vi "Execute.vi"(5 "Init user event out":refnum<user-event>, 7 "user event in":refnum<user-event>, 8 "Advanced Waveform In":refnum<class "Advanced Waveform.lvclass">, 9 "Generate From File in":refnum<class "Generate From File.lvclass">, 10 "Command Queue":refnum<queue>, 11 "error in (no error)":errorcluster) -> (0 "Advanced Waveform Out":refnum<class "Advanced Waveform.lvclass">, 1 "Generate From File Out":refnum<class "Generate From File.lvclass">, 2 "Stop":bool, 3 "error out":errorcluster)   [LabVIEW 2011, in "Generate From File.lvclass"]
uses:
  Generate From File.lvclass
  Advanced Waveform Class/Advanced Waveform.lvclass
  Message.lvclass
  Generate Class/Generate.lvclass
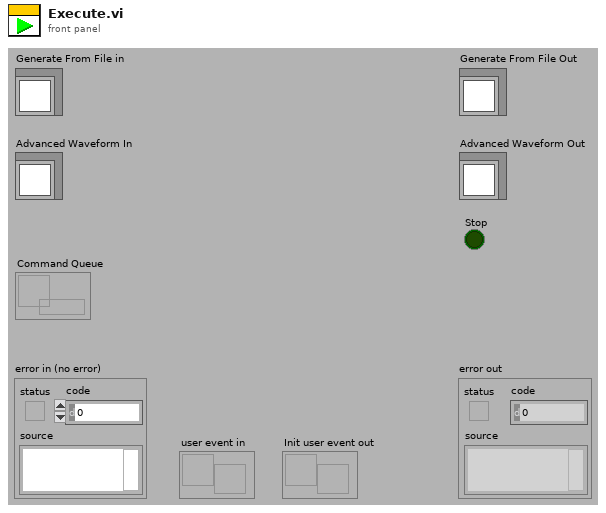
[diagram p1: front panel]
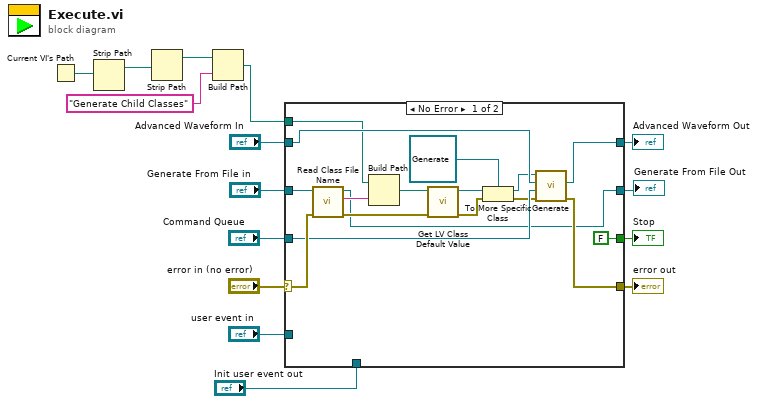
[diagram p0: block diagram]
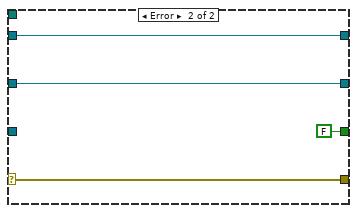
[diagram p2: hidden frame]
diagram:
  n1 = Current VI's Path() -> (path=w11:path)
  n2 = Strip Path(path=w11) -> (stripped path=w10:path)  [unwired: 1 out]
  n3 = Strip Path(path=w10) -> (stripped path=w9:path)  [unwired: 1 out]
  n4 = Build Path(base path=w9, name or relative path="Generate Child Classes") -> (appended path=w7:path)
  n5 = case shown="No Error" "error in (no error)" {
    selector: "error in (no error)" -> [w31 w35]
    tunnel: "Command Queue" -> [w26 _]
    tunnel: "Generate From File in" -> [w32 w33]
    tunnel: "Advanced Waveform In" -> [w28 w36]
    tunnel: w7 -> [w17 _]
    tunnel: [w27 w36] -> w6
    tunnel: [FALSE FALSE] -> w5
    tunnel: [w24 w35] -> w4
    tunnel: [w18 w33] -> w3
    tunnel: "user event in" -> [_ _]
    tunnel: "Init user event out" -> [_ _]
    frame No Error {
      n6 = call-dynamic "Read Class File Name.vi"("error in (no error)"=w31, "Generate From File in"=w32) -> ("error out"=w29:errorcluster, "Class File Name"=w30:string, "Generate From File out"=w18:refnum<class "Generate From File.lvclass">)  [unwired: 7 in]
      n7 = Build Path(base path=w17, name or relative path=w30) -> (appended path=w16:path)
      n8 = call <vilib>:"Get LV Class Default Value.vi"("error in (no error)"=w29, "class path"=w16) -> ("error out"=w22:errorcluster, "object"=w23:refnum<class>)  [unwired: 8 in]
      n9 = To More Specific Class(target class=refnum<class "Generate.lvclass"> refnum ("Generate.lvclass"), reference=w23, error in=w22) -> (specific class reference=w20:refnum<class "Generate.lvclass">, error out=w21:errorcluster)
      n10 = call-dynamic "Generate.vi"("error in (no error)"=w21, "Message Queue"=w26, "Advanced Waveform.lvclass In"=w28, "Generate in"=w20) -> ("error out"=w24:errorcluster, "Advanced Waveform.lvclass Out"=w27:refnum<class "Advanced Waveform.lvclass">)  [unwired: 4 in, 2 out]
    }
    frame Error {
    }
  }
  "error out" <- w4
  "Stop" <- w5
  "Advanced Waveform Out" <- w6
  "Generate From File Out" <- w3
